vi "Create Value.vi"(8 "error in":errorcluster, 11 "type code":T1=enum."AnyA") -> (0 "error out":errorcluster, 3 "value pointer out":i64)   [LabVIEW 2020, in "Value.lvlib"]
uses:
  Value.lvlib
  Type Code.ctl
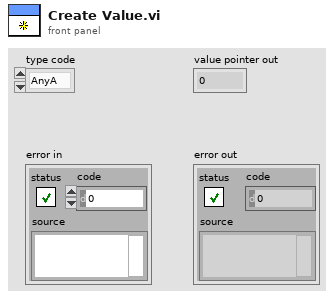
[diagram p1: front panel]
types:
  T1 = typedef "Value.lvlib/Type Code.ctl" = enum8{"Null", "Bool", "BoolA", "Int8", "Int8A", "Int16", "Int16A", "Int32", "Int32A", "Int64", "Int64A", "UInt8", "UInt8A", "UInt16", "UInt16A", "UInt32", "UInt32A", "UInt64", "UInt64A", "Float32", "Float32A", "Float64", "Float64A", "String", "StringA", "Struct", "StructA", "Union", "UnionA", "Any", "AnyA"}
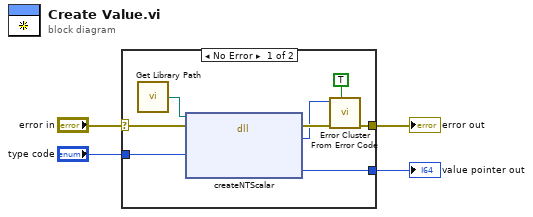
[diagram p0: block diagram]
diagram:
  n1 = case shown="No Error" "error in" {
    selector: "error in" -> [w11 w13]
    tunnel: [w7 w13] -> w4
    tunnel: [w6 _] -> w2
    tunnel: "type code" -> [w5 _]
    frame No Error {
      n2 = call "Get Library Path.vi"() -> ("Path"=w12:path)  [unwired: 1 in]
      n3 = dll-call lib="?" fn="createNTScalar"(path in=w12, error in=w11, "type_code"=w5) -> (error out=w9:errorcluster, "err_code"=w8:i32, "value"=w6:i64)  [unwired: 3 in, 1 out]
      n4 = call <vilib>:"Error Cluster From Error Code.vi"("show call chain? (False)"=TRUE, "error in (no error)"=w9, "error code (0)"=w8) -> ("error out"=w7:errorcluster)  [unwired: 6 in]
    }
    frame Error {
    }
  }
  "error out" <- w4
  "value pointer out" <- w2
